vi "Global FITS Path Variable.vi"() -> ()   [LabVIEW 2014]
panel:
  in  "Current FITS Path":path
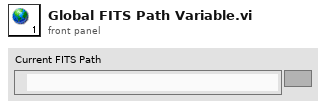
[diagram p1: front panel]
diagram:
